vi "Apply Filter.vi"   [LabVIEW 2015, in "E2E Tag Exchange editor node.lvclass"]
uses:
  E2E Tag Exchange editor node.lvclass
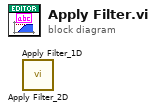
[diagram p0: block diagram]
diagram:
  n1 = call "Apply Filter_2D.vi"() -> ()  [unwired: 11 in, 1 out]
  n2 = call "Apply Filter_1D.vi"() -> ()  [unwired: 11 in, 1 out]
